vi "Remove Buffer.vi"(8 "error in":errorcluster, 9 "Name":string, 11 "BufferMap in":refnum<data-value>) -> (0 "error out":errorcluster, 2 "Buffer":refnum<data-value>, 3 "BufferMap":refnum<data-value>)   [LabVIEW 2013, in "CircularBuffer.lvlib" / "VariantBufferMap.lvclass"]
doc: "This VI writes one data element into the current location in the buffer. The location in the buffer is updated automatically."
uses:
  VariantBufferMap.lvclass
  VariantBuffer/VariantBuffer.lvclass
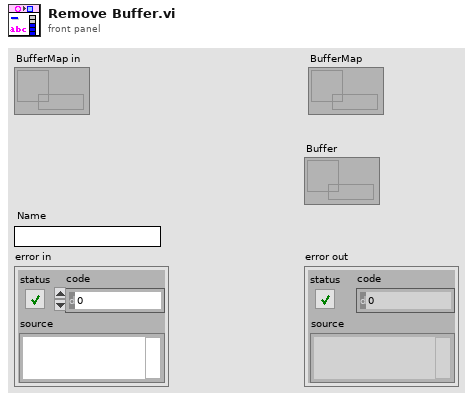
[diagram p1: front panel]
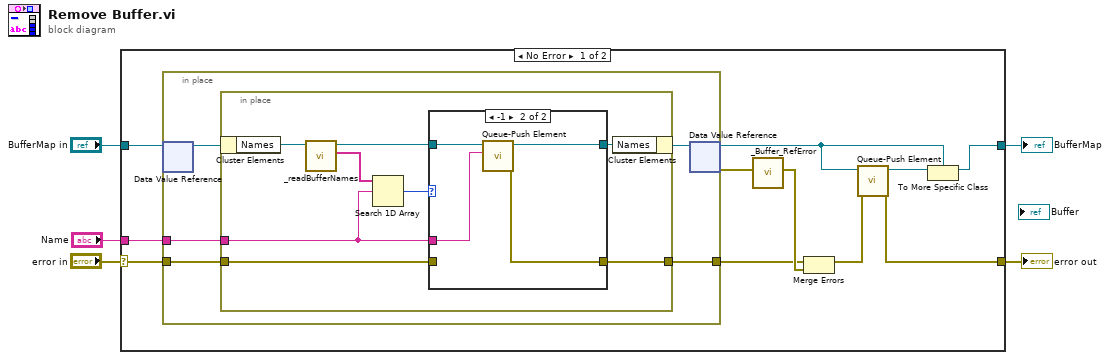
[diagram p0: block diagram]
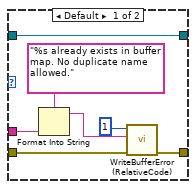
[diagram p2: hidden frame]
diagram:
  n1 = case shown="No Error" "error in" {
    selector: "error in" -> [w8 w42]
    tunnel: "BufferMap in" -> [w13 w41]
    tunnel: [w14 w41] -> w4
    tunnel: [w9 w42] -> w3
    tunnel: "Name" -> [w16 _]
    frame No Error {
      n2 = in-place {
        in-place-border: w16 -> [w19]
        in-place-border: [w18] -> w7
        in-place-border: w8 -> [w17]
        n3 = in-place-dvr #1(w13) -> (w21:refnum<class "VariantBufferMap.lvclass">)  [unwired: 1 out]
        n4 = in-place {
          in-place-border: w19 -> [w27]
          in-place-border: [w26] -> w18
          in-place-border: w17 -> [w22]
          n5 = in-place-cluster #2(w21) -> ("Names"=w29:refnum<data-value>)
          n6 = call "_readBufferNames.vi"("Data Value Reference in"=w29) -> ("Names"=w25:string[], "Data Value Reference out"=w23:refnum<data-value>)  [unwired: 9 in]
          n7 = Search 1D Array(1D array=w25, element=w27) -> (index of element=w24:i32)  [unwired: 1 in]
          n8 = case shown="-1" w24 {
            tunnel: w23 -> [w36 w40]
            tunnel: [w36 w39] -> w28
            tunnel: w27 -> [w32 w37]
            tunnel: [w35 w38] -> w26
            tunnel: w22 -> [w33 _]
            frame Default {
              n9 = Format Into String(format string="%s already exists in buffer map. No duplicate name allowed." ("error message (\"\")"), w32) -> (resulting string=w31:string)  [unwired: 2 in, 1 out]
              n10 = call "WriteBufferError (RelativeCode).vi"("error in (no error)"=w33, "Error message"=w31, "Relative error code (548600 + input)"=1 ("error code (0)")) -> ("error out"=w35:errorcluster)  [unwired: 8 in]
            }
            frame -1 {
              n11 = call "Queue-Push Element.vi"("element"=w37, "Buffer in"=w40) -> ("error out"=w38:errorcluster, "Buffer"=w39:refnum<data-value>)  [unwired: 6 in, 2 out]
            }
          }
          n12 = in-place-cluster #2("Names"=w28) -> (w20:refnum<class "VariantBufferMap.lvclass">)
        }
        n13 = in-place-dvr #1(w20) -> (w6:refnum<data-value>, w12:errorcluster)
      }
      n14 = call "_Buffer_RefError.vi"("error in (no error)"=w12) -> ("error out"=w11:errorcluster)  [unwired: 10 in]
      n15 = Merge Errors(w7, w11) -> (w10:errorcluster)
      n16 = call "Queue-Push Element.vi"("error in"=w10, "Buffer in"=w6) -> ("error out"=w9:errorcluster, "Buffer"=w15:refnum<data-value>)  [unwired: 6 in, 2 out]
      n17 = To More Specific Class(target class=w6, reference=w15) -> (specific class reference=w14:refnum<data-value>)  [unwired: 1 in, 1 out]
    }
    frame Error {
    }
  }
  "error out" <- w3
  "BufferMap" <- w4
